vi "rc_get state.vi"(8 "error in (no error)":errorcluster) -> (0 "error out":errorcluster, 3 "function return":u32(ring))   [LabVIEW 2014, in "libroboticscape.lvlib"]
doc: "state_t get_state();"
uses:
  libroboticscape.lvlib
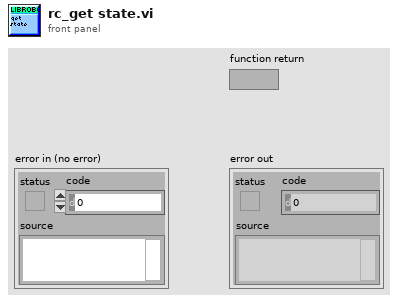
[diagram p1: front panel]
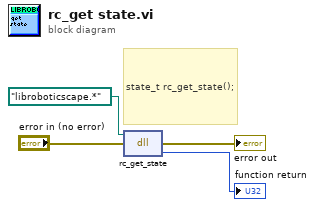
[diagram p0: block diagram]
diagram:
  # "state_t rc_get_state();"
  n1 = dll-call lib="C:/Users/ktalke/Documents/Robotics-Cape-Master-Jessie/Libroboticscape-Master-Jessie/libroboticscape.so" fn="rc_get_state"(path in=path "libroboticscape.*", error in="error in (no error)") -> (error out=→"error out":errorcluster, "return type"=→"function return":u32)  [unwired: 1 in, 1 out]
